vi "ratio.vi"(11 "Numeric in":dbl) -> (3 "Numeric out":dbl)   [LabVIEW 2020]
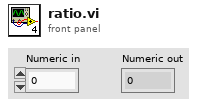
[diagram p1: front panel]
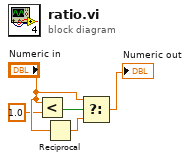
[diagram p0: block diagram]
diagram:
  n1 = Less?(x="Numeric in", y=1.0) -> (x < y?=w2:bool)
  n2 = Reciprocal(x="Numeric in") -> (1/x=w4:dbl)
  n3 = Select(t="Numeric in", s=w2, f=w4) -> (s? t:f=→"Numeric out":dbl)
